vi "varXNode_Compare.vi"(4 "Data In":T2, 5 "State In":T2) -> (2 "Diffs":T1(array[cluster]))   [LabVIEW 2020, in "varXNode.xnode"]
uses:
  <vilib>/variable/varXNode.llb/varXNode.xnode
  <vilib>/variable/varXNode.llb/varXNode.ctl
  <vilib>/variable/Type Descriptor.ctl
  <vilib>/variable/NI_Variable.lvlib
panel:
  # "Major = True,\nMinor = False"
  # "Functional = True,\nCosmetic = False"
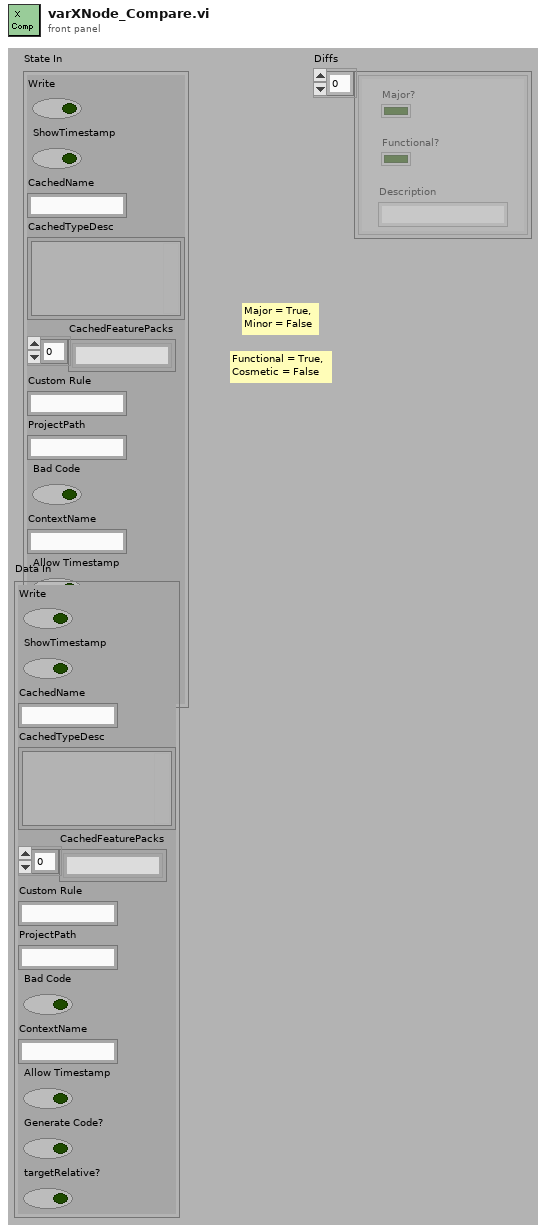
[diagram p1: front panel]
types:
  T1 = cluster{"Description":string, "Major?":bool, "Functional?":bool}[]
  T2 = typedef "varXNode.xnode/varXNode.ctl" = cluster{"Write":bool, "ShowTimestamp":bool, "CachedName":string, "CachedTypeDesc":T3, "CachedFeaturePacks":string[], "Custom Rule":string, "ProjectPath":string, "Bad Code":bool, "ContextName":string, "Allow Timestamp":bool, "Generate Code?":bool, "targetRelative?":bool}
  T3 = typedef "NI_Variable.lvlib/Type Descriptor.ctl" = cluster{"Variant":variant}
  T4 = cluster{"Description":string, "Major?":bool, "Functional?":bool}
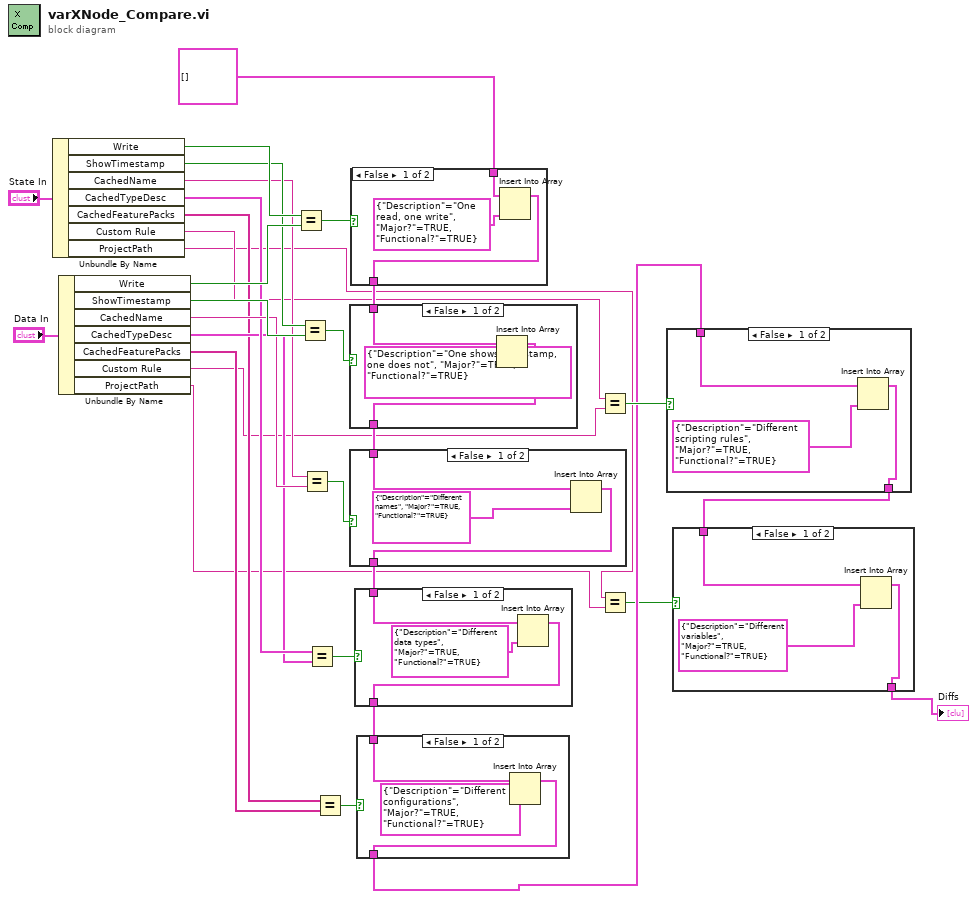
[diagram p0: block diagram]
diagram:
  n1 = Unbundle By Name("State In") -> ("Write"=w29:bool, "ShowTimestamp"=w25:bool, "CachedName"=w21:string, "CachedTypeDesc"=w15:T3, "CachedFeaturePacks"=w11:string[], "Custom Rule"=w8:string, "ProjectPath"=w2:string)
  n2 = Unbundle By Name("Data In") -> ("Write"=w28:bool, "ShowTimestamp"=w24:bool, "CachedName"=w20:string, "CachedTypeDesc"=w14:T3, "CachedFeaturePacks"=w10:string[], "Custom Rule"=w7:string, "ProjectPath"=w1:string)
  n3 = Equal?(x=w29, y=w28) -> (x = y?=w27:bool)
  n4 = Equal?(x=w25, y=w24) -> (x = y?=w23:bool)
  n5 = Equal?(x=w21, y=w20) -> (x = y?=w19:bool)
  n6 = Equal?(x=w15, y=w14) -> (x = y?=w16:bool)
  n7 = Equal?(x=w11, y=w10) -> (x = y?=w12:bool)
  n8 = case shown="False" w27 {
    tunnel: T1 [] ("Diffs") -> [w34 w35]
    tunnel: [w32 w35] -> w22
    frame False {
      n9 = Insert Into Array(array=w34, new element=T4 {"Description"="One read, one write", "Major?"=TRUE, "Functional?"=TRUE} ("Diff")) -> (w32:T1)  [unwired: 1 in]
    }
    frame True {
    }
  }
  n10 = case shown="False" w23 {
    tunnel: w22 -> [w37 w39]
    tunnel: [w36 w39] -> w18
    frame False {
      n11 = Insert Into Array(array=w37, new element=T4 {"Description"="One shows timestamp, one does not", "Major?"=TRUE, "Functional?"=TRUE} ("Diff")) -> (w36:T1)  [unwired: 1 in]
    }
    frame True {
    }
  }
  n12 = case shown="False" w19 {
    tunnel: w18 -> [w41 w43]
    tunnel: [w40 w43] -> w17
    frame False {
      n13 = Insert Into Array(array=w41, new element=T4 {"Description"="Different names", "Major?"=TRUE, "Functional?"=TRUE} ("Diff")) -> (w40:T1)  [unwired: 1 in]
    }
    frame True {
    }
  }
  n14 = case shown="False" w16 {
    tunnel: w17 -> [w45 w47]
    tunnel: [w44 w47] -> w13
    frame False {
      n15 = Insert Into Array(array=w45, new element=T4 {"Description"="Different data types", "Major?"=TRUE, "Functional?"=TRUE} ("Diff")) -> (w44:T1)  [unwired: 1 in]
    }
    frame True {
    }
  }
  n16 = case shown="False" w12 {
    tunnel: w13 -> [w49 w51]
    tunnel: [w48 w51] -> w6
    frame False {
      n17 = Insert Into Array(array=w49, new element=T4 {"Description"="Different configurations", "Major?"=TRUE, "Functional?"=TRUE} ("Diff")) -> (w48:T1)  [unwired: 1 in]
    }
    frame True {
    }
  }
  n18 = Equal?(x=w8, y=w7) -> (x = y?=w9:bool)
  n19 = Equal?(x=w2, y=w1) -> (x = y?=w3:bool)
  n20 = case shown="False" w9 {
    tunnel: w6 -> [w54 w55]
    tunnel: [w53 w55] -> w5
    frame False {
      n21 = Insert Into Array(array=w54, new element=T4 {"Description"="Different scripting rules", "Major?"=TRUE, "Functional?"=TRUE} ("Diff")) -> (w53:T1)  [unwired: 1 in]
    }
    frame True {
    }
  }
  n22 = case shown="False" w3 {
    tunnel: w5 -> [w58 w59]
    tunnel: [w57 w59] -> w4
    frame False {
      n23 = Insert Into Array(array=w58, new element=T4 {"Description"="Different variables", "Major?"=TRUE, "Functional?"=TRUE} ("Diff")) -> (w57:T1)  [unwired: 1 in]
    }
    frame True {
    }
  }
  "Diffs" <- w4
